vi "MCP3208 I2C Analog Input.vi"   [LabVIEW 2014]
uses:
  QwaveSys_Interface/QwaveSys_Interface.lvlib
  QwaveSys_ESP8266/QwaveSys_ESP8266.lvlib
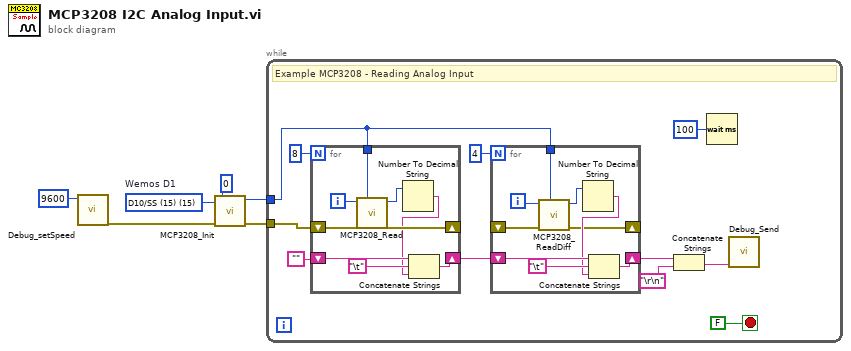
[diagram p0: block diagram]
diagram:
  w3 = u8 15 items=["D0-RX(3)"=3, "D1-TX(1)"=1, "D2(16)"=16, "D3/D15/SCL(5)"=5, "D4/D14/SDA(4)"=4, "D5/D13/SCK(14)-(LED)"=14, "D6/D12/MISO(12)"=12, "D7/D11/MOSI(13)"=13, "D8(0)"=0, "D9/TX1(2)"=2, "D10/SS (15)"=15, "ADC0,(17)"=17]  # Wemos D1
  n1 = call "Debug_setSpeed.vi"("Speed"=u32 9600) -> ("error out"=w2:errorcluster)  [unwired: 10 in]
  n2 = call "MCP3208_Init.vi"("error in"=w2, "CS"=w3, "Interface (0-4)"=u8 0) -> ("error out"=w4:errorcluster, "Instance"=w5:u8)  [unwired: 7 in]
  n3 = while {
    tunnel: w5 -> [w11]
    tunnel: w4 -> [w17]
    stop <- FALSE stop-if-true
    # "Example MCP3208 - Reading Analog Input"
    n4 = for {
      N: 8 -> [_]
      shift-right: [w34] -> _
      shift-left: w17 -> [w35]
      shift-right: [w32] -> w10
      shift-left: "" ("Empty String Constant") -> [w31]
      tunnel: w11 -> [w27]
      i -> [w33]
      n5 = call "MCP3208_Read.vi"("Instance"=w27, "error in (no error)"=w35, "Channel (0-7)"=w33) -> ("error out"=w34:errorcluster, "ADC"=w29:u16)  [unwired: 7 in]
      n6 = Number To Decimal String(number=w29) -> (decimal integer string=w28:string)  [unwired: 1 in]
      n7 = Concatenate Strings(w31, "\t" ("Tab Constant"), w28) -> (w32:string)
    }
    n8 = for {
      N: 4 -> [_]
      shift-right: [w21] -> _
      shift-left: _ -> [w22]
      shift-right: [w26] -> w9
      shift-left: w10 -> [w25]
      tunnel: w11 -> [w19]
      i -> [w20]
      n9 = call "MCP3208_ReadDiff.vi"("Instance"=w19, "error in (no error)"=w22, "Channel (0-3)"=w20) -> ("error out"=w21:errorcluster, "Ch Diff ADC"=w18:i16)  [unwired: 7 in]
      n10 = Number To Decimal String(number=w18) -> (decimal integer string=w23:string)  [unwired: 1 in]
      n11 = Concatenate Strings(w25, "\t" ("Tab Constant"), w23) -> (w26:string)
    }
    n12 = Concatenate Strings(w9, "\r\n" ("End of Line Constant")) -> (w7:string)
    n13 = Wait (ms)(milliseconds to wait=u32 100) -> ()  [unwired: 1 out]
    n14 = call "Debug_Send.vi"("DATA"=w7) -> ()  [unwired: 11 in]
  }
